vi "main.vi"(0 "File Name":string="log.txt" caption="File Name (without extension)", 1 "Count_size":i32=1 min=1 step=1, 5 "File size":i64=100 min=10, 7 "Maximum":u64=1 min=1 max=100 step=1, 9 "Minimum":u64=1 min=1 max=100 step=1, 11 "error constant":errorcluster) -> (6 "Moving average":dbl(graph), 15 "error out":errorcluster)   [LabVIEW 2023, in "task-1.lvlib"]
uses:
  controls/Operations.ctl
  task-1.lvlib
panel:
  in  "Stop":bool
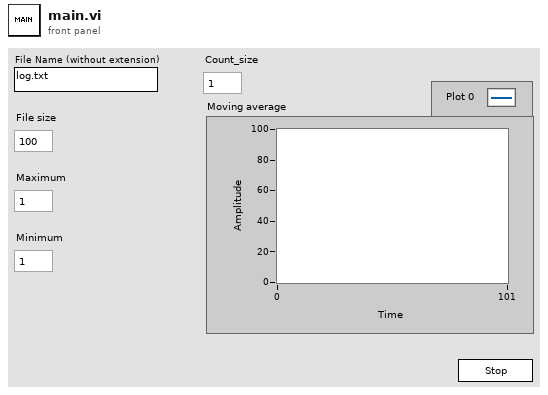
[diagram p1: front panel]
types:
  T1 = typedef "task-1.lvlib/Operations.ctl" = enum16{"Set_Stop", "Get_array", "Get_last_val", "Add_val", "Initialize"}
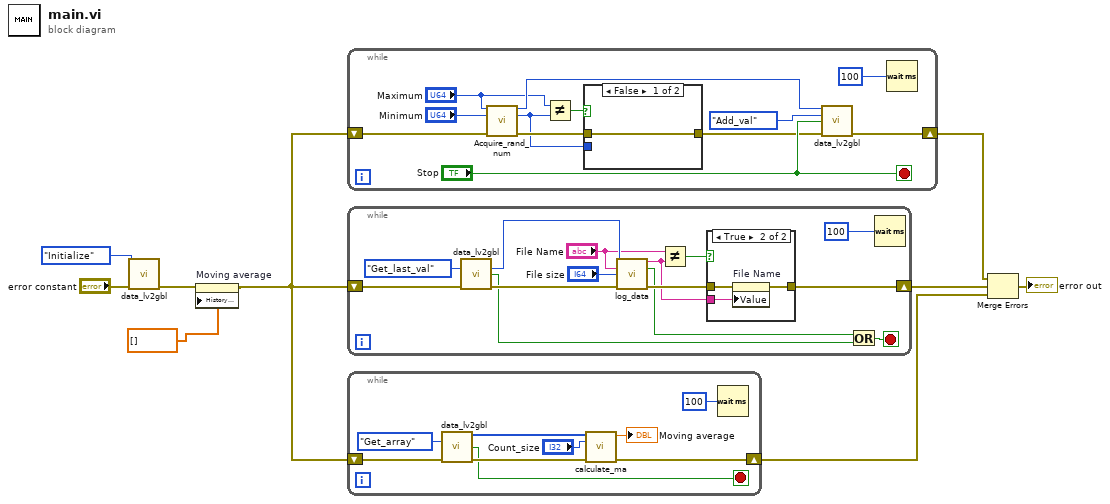
[diagram p0: block diagram]
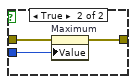
[diagram p3: hidden frame]
diagram:
  n1 = call "data_lv2gbl.vi"("Operations"=Operations."Initialize", "error in"="error constant") -> ("error out"=w3:errorcluster)  [unwired: 10 in, 3 out]
  n2 = property on="Moving average" class="WFChart (strict)"(error in=w3, "History Data"=dbl[] []) -> (error out=w2:errorcluster)  [unwired: 1 in, 1 out]
  n3 = while {
    shift-right: [w18] -> w9
    shift-left: w2 -> [w19]
    stop <- "Stop" stop-if-true
    n4 = call "Acquire_rand_num.vi"("Upper limit"="Maximum", "Lower limit"="Minimum", "error in"=w19) -> ("Data"=w16:u64, "Coerce upper"=w10:u64, "error out"=w14:errorcluster)  [unwired: 10 in]
    n5 = Not Equal?(x="Maximum", y=w10) -> (x != y?=w12:bool)
    n6 = case shown="False" w12 {
      tunnel: w14 -> [w22 w25]
      tunnel: [w22 w24] -> w13
      tunnel: w10 -> [_ w23]
      frame False {
      }
      frame True {
        n7 = property on="Maximum" class="DigNum (strict)"(error in=w25, "Value"=w23) -> (error out=w24:errorcluster)  [unwired: 1 in, 1 out]
      }
    }
    n8 = call "data_lv2gbl.vi"("Data"=w16, "Operations"=Operations."Add_val", "Stop_in"="Stop", "error in"=w13) -> ("error out"=w18:errorcluster)  [unwired: 8 in, 3 out]
    n9 = Wait (ms)(milliseconds to wait=u32 100) -> ()  [unwired: 1 out]
  }
  n10 = while {
    shift-right: [w29] -> w7
    shift-left: w2 -> [w37]
    stop <- w28 stop-if-true
    n11 = call "data_lv2gbl.vi"("Operations"=Operations."Get_last_val", "error in"=w37) -> ("Last_val"=w35:u64, "Stop_out"=w27:bool, "error out"=w36:errorcluster)  [unwired: 10 in, 1 out]
    n12 = call "log_data.vi"("Data"=w35, "File Name"="File Name", "File size(kb)"="File size", "error in"=w36) -> ("File Name out"=w30:string, "Stop_logging"=w26:bool, "error out"=w31:errorcluster)  [unwired: 9 in]
    n13 = Not Equal?(x="File Name", y=w30) -> (x != y?=w32:bool)
    n14 = case shown="True" w32 {
      tunnel: w31 -> [w40 w43]
      tunnel: [w40 w42] -> w29
      tunnel: w30 -> [_ w41]
      frame False {
      }
      frame True {
        n15 = property on="File Name" class="Str"(error in=w43, "Value"=w41) -> (error out=w42:errorcluster)  [unwired: 1 in, 1 out]
      }
    }
    n16 = Or(x=w26, y=w27) -> (x .or. y?=w28:bool)
    n17 = Wait (ms)(milliseconds to wait=u32 100) -> ()  [unwired: 1 out]
  }
  n18 = while {
    shift-right: [w51] -> w6
    shift-left: w2 -> [w48]
    stop <- w45 stop-if-true
    n19 = call "data_lv2gbl.vi"("Operations"=Operations."Get_array", "error in"=w48) -> ("Data out"=w44:u64[], "Stop_out"=w45:bool, "error out"=w47:errorcluster)  [unwired: 10 in, 1 out]
    n20 = call "calculate_ma.vi"("Data_points"=w44, "Count_size"="Count_size", "error in"=w47) -> ("Cur_avg"=→"Moving average":dbl, "error out"=w51:errorcluster)  [unwired: 11 in]
    n21 = Wait (ms)(milliseconds to wait=u32 100) -> ()  [unwired: 1 out]
  }
  n22 = Merge Errors(w9, w7, w6) -> (→"error out":errorcluster)
